vi "mapV5.vi"() -> ()   [LabVIEW 2024]
uses:
  D:/Autonomous Systems/Oulu/Measurment Systems/EnvironmentalMonitoringSystem/GMapControl/GMapControl/bin/Debug/GMapControl.dll
  GMapControl/GMapControl/bin/Debug/GMapControl.dll
  C:/Program Files (x86)/National Instruments/LabVIEW 2024/examples/Design Patterns/Queued Message Handler/support/QMH Fundamentals - Message Cluster.ctl
  API_Key.vi
  isMapRun.vi
panel:
  out "API_key_delievered":bool=TRUE
  out "GetLastAction":i32
  out "id_list":u16[](array[numeric])
  out "GetLongitude":dbl
  out "GetLatitude":dbl
  out "Button":u16
  out "mouse event":bool
  in  "MapControl":refnum<k24>(container)
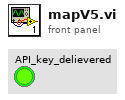
[diagram p1: front panel]
types:
  T1 = typedef "QMH Fundamentals - Message Cluster.ctl" = cluster{"Message":string, "Message Data":variant}
  T2 = cluster{"meta":cluster{"name":string, "website":string, "page":dbl, "limit":dbl}, "results":cluster{"id":i32, "name":string, "distance":dbl, "coordinates":cluster{"latitude":dbl, "longitude":dbl}}[]}
  T3 = cluster{"id":i32, "name":string, "distance":dbl, "coordinates":cluster{"latitude":dbl, "longitude":dbl}}[]
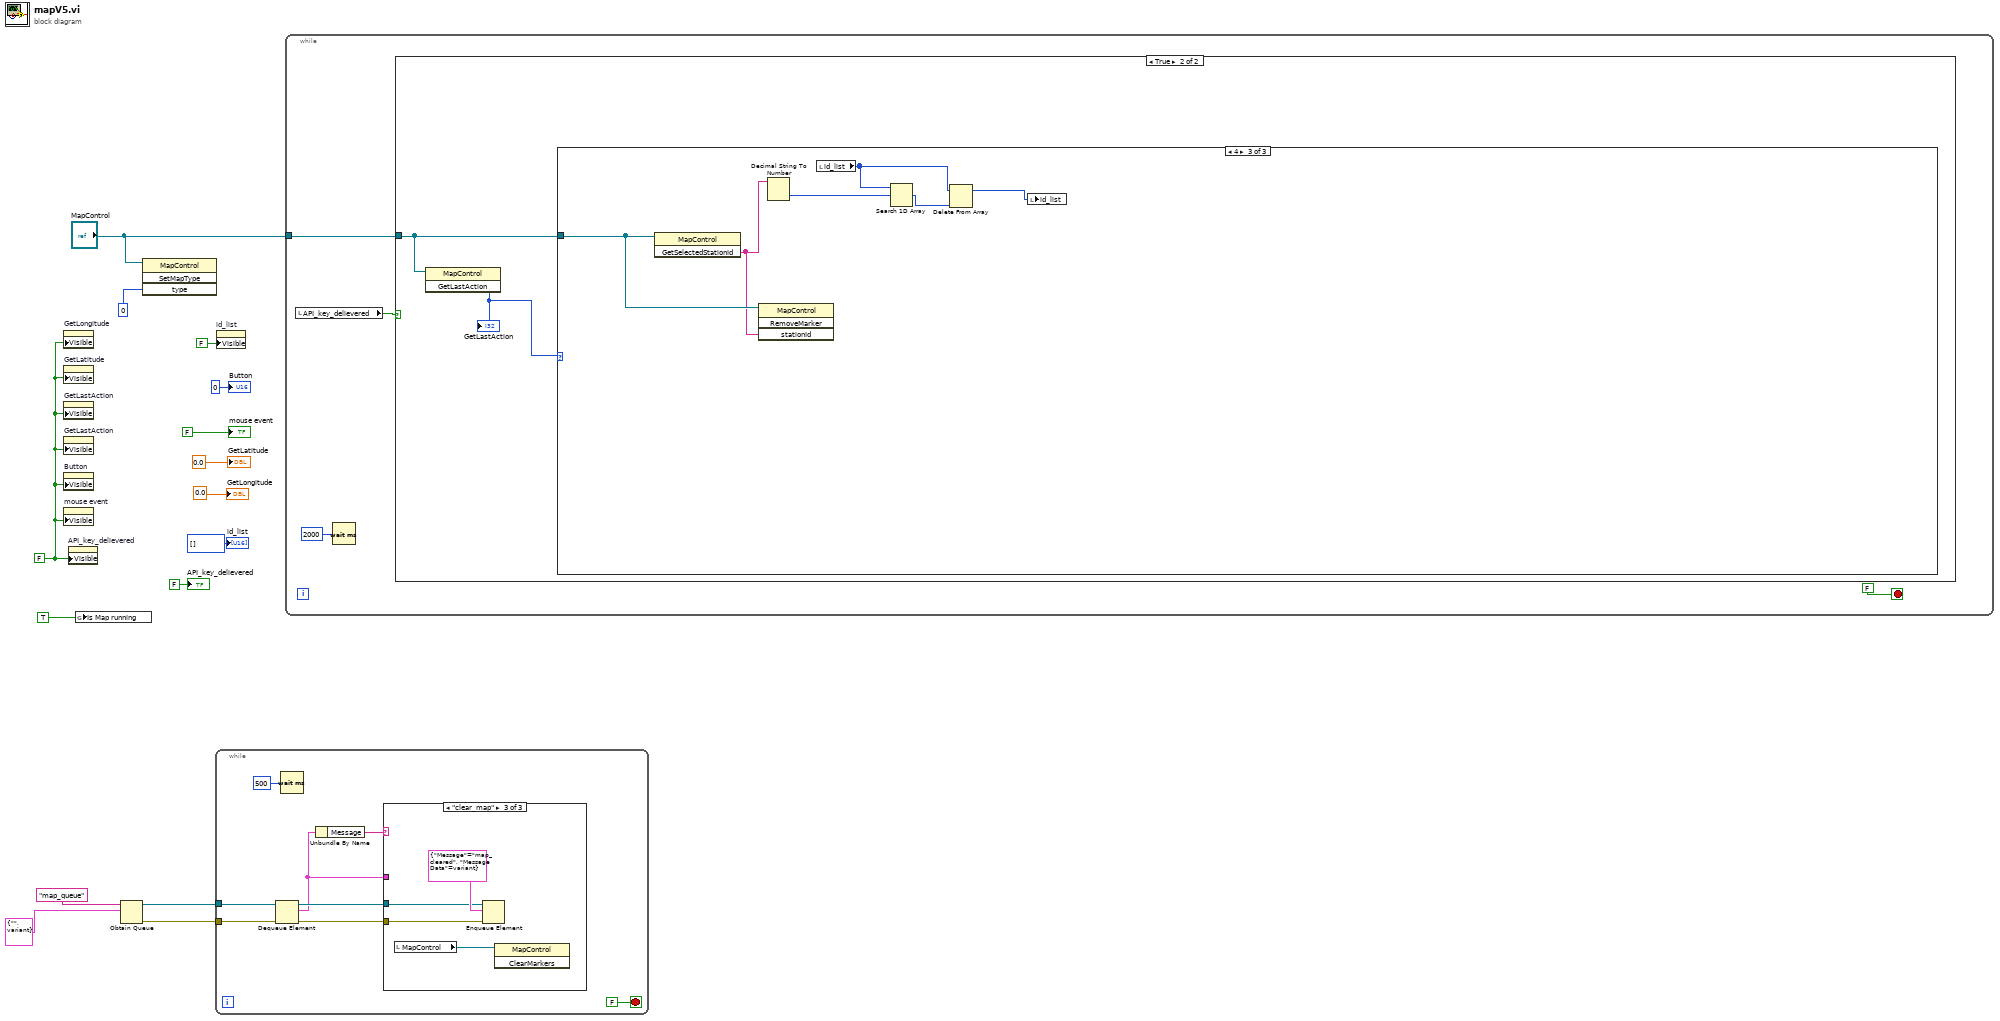
[diagram p0: block diagram]
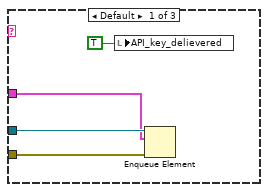
[diagram p2: hidden frame]
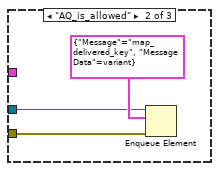
[diagram p3: hidden frame]
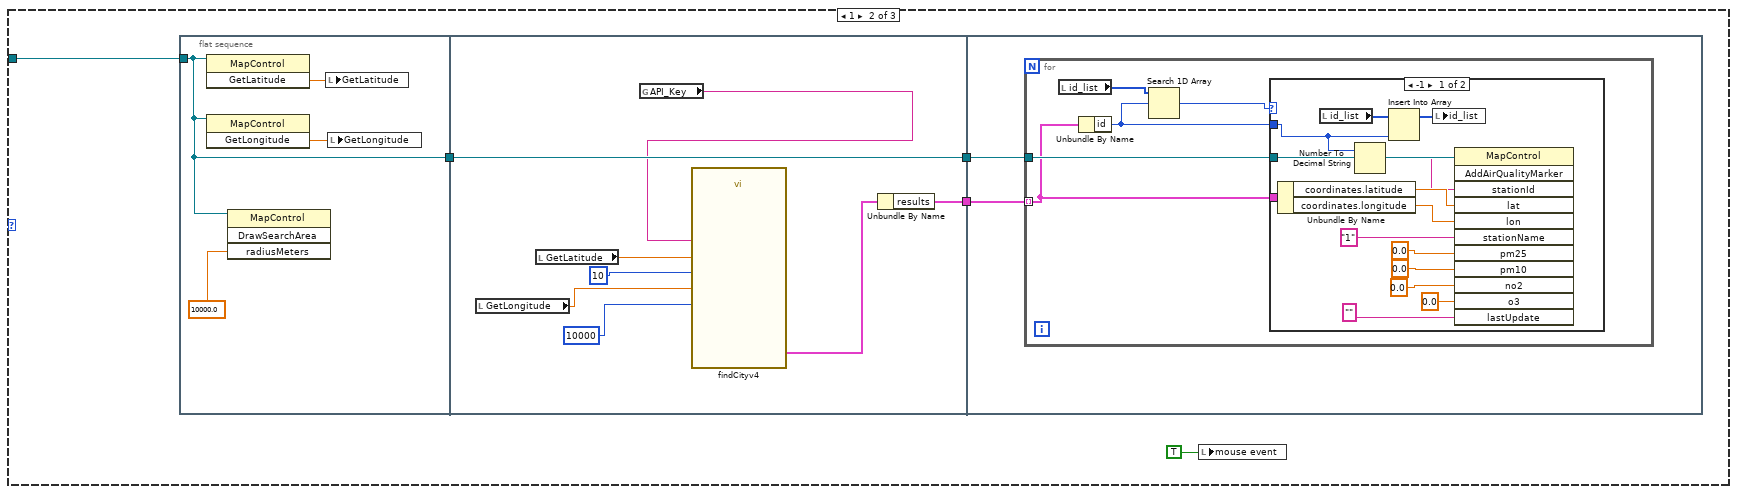
[diagram p6: hidden frame]
diagram:
  w2 = FALSE ("Visible")
  n1 = property on="GetLongitude" class="DigNum (strict)"("Visible"=w2) -> ()  [unwired: 2 in, 2 out]
  n2 = property on="GetLatitude" class="DigNum (strict)"("Visible"=w2) -> ()  [unwired: 2 in, 2 out]
  n3 = property on="GetLastAction" class="DigNum (strict)"("Visible"=w2) -> ()  [unwired: 2 in, 2 out]
  n4 = property on="GetLastAction" class="DigNum (strict)"("Visible"=w2) -> ()  [unwired: 2 in, 2 out]
  n5 = property on="Button" class="DigNum (strict)"("Visible"=w2) -> ()  [unwired: 2 in, 2 out]
  n6 = property on="mouse event" class="Bool (strict)"("Visible"=w2) -> ()  [unwired: 2 in, 2 out]
  n7 = property on="API_key_delievered" class="Bool (strict)"("Visible"=w2) -> ()  [unwired: 2 in, 2 out]
  n8 = global write "isMapRun.vi" "Is Map running"(TRUE ("Is Map running")) -> ()
  n9 = Obtain Queue(name (unnamed)="map_queue", element data type=T1 {"Message"="", "Message Data"=variant} ("Message Cluster")) -> (queue out=w5:refnum<queue>, error out=w4:errorcluster)  [unwired: 3 in, 1 out]
  n10 = invoke class="MapControl" method="SetMapType"(reference="MapControl", "type"=0) -> ()  [unwired: 2 in, 4 out]
  n11 = while {
    tunnel: w5 -> [w23]
    tunnel: w4 -> [w22]
    stop <- FALSE stop-if-true
    n12 = Dequeue Element(queue=w23, error in (no error)=w22) -> (queue out=w18:refnum<queue>, element=w16:T1, error out=w17:errorcluster)  [unwired: 1 in, 1 out]
    n13 = Wait (ms)(milliseconds to wait=u32 500) -> ()  [unwired: 1 out]
    n14 = Unbundle By Name(w16) -> ("Message"=w20:string)
    n15 = case shown="\"clear_map\"" w20 {
      tunnel: w18 -> [w27 w29 w33]
      tunnel: w17 -> [w26 w28 w32]
      tunnel: w16 -> [w25 _ _]
      frame Default {
        n16 = local write "API_key_delievered"(TRUE ("API_key_delievered")) -> ()
        n17 = Enqueue Element(queue=w27, element=w25, error in (no error)=w26) -> ()  [unwired: 1 in, 3 out]
      }
      frame "AQ_is_allowed" {
        n18 = Enqueue Element(queue=w29, element=T1 {"Message"="map_delivered_key", "Message Data"=variant}, error in (no error)=w28) -> ()  [unwired: 1 in, 3 out]
      }
      frame "clear_map" {
        n19 = local read "MapControl"() -> (w31:refnum<k24>)
        n20 = Enqueue Element(queue=w33, element=T1 {"Message"="map_cleared", "Message Data"=variant}, error in (no error)=w32) -> ()  [unwired: 1 in, 3 out]
        n21 = invoke class="MapControl" method="ClearMarkers"(reference=w31) -> ()  [unwired: 2 in, 3 out]
      }
    }
  }
  n22 = property on="id_list" class="Arr (strict)"("Visible"=FALSE) -> ()  [unwired: 2 in, 2 out]
  n23 = while {
    tunnel: "MapControl" -> [w36]
    stop <- FALSE stop-if-true
    n24 = local read "API_key_delievered"() -> (w35:bool)
    n25 = Wait (ms)(milliseconds to wait=u32 2000) -> ()  [unwired: 1 out]
    n26 = case shown="True" w35 {
      tunnel: w36 -> [_ w40]
      frame False {
      }
      frame True {
        n27 = invoke class="MapControl" method="GetLastAction"(reference=w40) -> ("GetLastAction"=w39:i32)  [unwired: 2 in, 2 out]
        "GetLastAction" <- w39
        n28 = case shown="4" w39 {
          tunnel: w40 -> [_ w45 w84]
          frame Default {
          }
          frame 1 {
            n29 = flat-sequence {
              tunnel: [w47] -> w43
              tunnel: w45 -> [w47]
              tunnel: w43 -> [w57]
              tunnel: [w57] -> w42
              tunnel: [w56] -> w41
              tunnel: w42 -> [w59]
              tunnel: w41 -> [w58]
              frame #0 {
                n30 = invoke class="MapControl" method="GetLatitude"(reference=w47) -> ("GetLatitude"=w49:dbl)  [unwired: 2 in, 2 out]
                n31 = invoke class="MapControl" method="GetLongitude"(reference=w47) -> ("GetLongitude"=w48:dbl)  [unwired: 2 in, 2 out]
                n32 = invoke class="MapControl" method="DrawSearchArea"(reference=w47, "radiusMeters"=10000.0) -> ()  [unwired: 2 in, 4 out]
                n33 = local write "GetLatitude"(w49) -> ()
                n34 = local write "GetLongitude"(w48) -> ()
              }
              frame #1 {
                n35 = local read "GetLongitude"() -> (w53:dbl)
                n36 = local read "GetLatitude"() -> (w55:dbl)
                n37 = global read "API_Key.vi" "API_Key"() -> (w50:string)
                n38 = call "findCityv4.vi"("limit"=u16 10, "API-key"=w50, "longitude"=w53, "latitude"=w55, "range"=u16 10000) -> ("value"=w51:T2)  [unwired: 2 out]
                n39 = Unbundle By Name(w51) -> ("results"=w56:T3)
              }
              frame #2 {
                n40 = for {
                  tunnel: w59 -> [w64]
                  tunnel: w58 -> [w60] mode=indexing
                  n41 = local read "id_list"() -> (w63:u16[])
                  n42 = Unbundle By Name(w60) -> ("id"=w61:i32)
                  n43 = Search 1D Array(1D array=w63, element=w61) -> (index of element=w62:i32)  [unwired: 1 in]
                  n44 = case shown="-1" w62 {
                    tunnel: w64 -> [w78 _]
                    tunnel: w60 -> [w75 _]
                    tunnel: w61 -> [w66 _]
                    frame -1 {
                      n45 = Unbundle By Name(w75) -> ("coordinates.latitude"=w67:dbl, "coordinates.longitude"=w68:dbl)
                      n46 = local read "id_list"() -> (w73:u16[])
                      n47 = Number To Decimal String(number=w66) -> (decimal integer string=w65:string)  [unwired: 1 in]
                      n48 = Insert Into Array(array=w73, new element=w66) -> (w74:u16[])  [unwired: 1 in]
                      n49 = local write "id_list"(w74) -> ()
                      n50 = invoke class="MapControl" method="AddAirQualityMarker"(reference=w78, "stationId"=w65, "lat"=w67, "lon"=w68, "stationName"="1", "pm25"=0.0 ("pm10"), "pm10"=0.0 ("no2"), "no2"=0.0 ("o3"), "o3"=0.0, "lastUpdate"="") -> ()  [unwired: 2 in, 12 out]
                    }
                    frame Default {
                    }
                  }
                }
              }
            }
            n51 = local write "mouse event"(TRUE ("mouse event")) -> ()
          }
          frame 4 {
            n52 = invoke class="MapControl" method="GetSelectedStationId"(reference=w84) -> ("GetSelectedStationId"=w83:string)  [unwired: 2 in, 2 out]
            n53 = invoke class="MapControl" method="RemoveMarker"(reference=w84, "stationId"=w83) -> ()  [unwired: 2 in, 4 out]
            n54 = Decimal String To Number(string=w83) -> (number=w82:i32)  [unwired: 2 in, 1 out]
            n55 = local read "id_list"() -> (w81:u16[])
            n56 = Search 1D Array(1D array=w81, element=w82) -> (index of element=w80:i32)  [unwired: 1 in]
            n57 = Delete From Array(array=w81, index=w80) -> (array with subset deleted=w79:u16[])  [unwired: 1 in, 1 out]
            n58 = local write "id_list"(w79) -> ()
          }
        }
      }
    }
  }
  "mouse event" <- FALSE ("mouse event")
  "Button" <- u16 0 ("Button")
  "GetLatitude" <- 0.0 ("GetLatitude")
  "GetLongitude" <- 0.0 ("GetLongitude")
  "id_list" <- u16[] [] ("id_list")
  "API_key_delievered" <- FALSE ("Boolean")
